vi "NavX_MAIN_2.vi"() -> ()   [LabVIEW 2018]
uses:
  Underlying VI's/NavX VI/navX type def.ctl
  <vilib>/Studica/Studica Toolkit/NavX/TypeDefs/Flags/Z900_navX_Flags_OpStatusTypeDef.ctl
  <vilib>/Studica/Studica Toolkit/NavX/TypeDefs/Flags/Z900_navX_Flags_CalibrationStatusTypeDef.ctl
  <vilib>/Studica/Studica Toolkit/Background/I2C Channel.ctl
  <vilib>/Studica/Studica Toolkit/NavX/NavX.lvlib
panel:
  out "Error Out":errorcluster
  out "Status":T3 {"OP Status" items=["INITIALIZING", "SELFTEST_IN_PROGRESS", "ERROR", "IMU_AUTOCAL_IN_PROGRESS", "NORMAL"]; "Calibration Status" items=["IMU_CAL_STATE_MASK"=3, "IMU_CAL_STATE_INPROGRESS"=0, "IMU_CAL_STATE_ACCUMULATE"=1, "IMU_CAL_STATE_COMPLETE"=2]}
  out "NavX Readings":T4
  in  "Mode":T5=enum."Read Values"
  in  "stop":bool
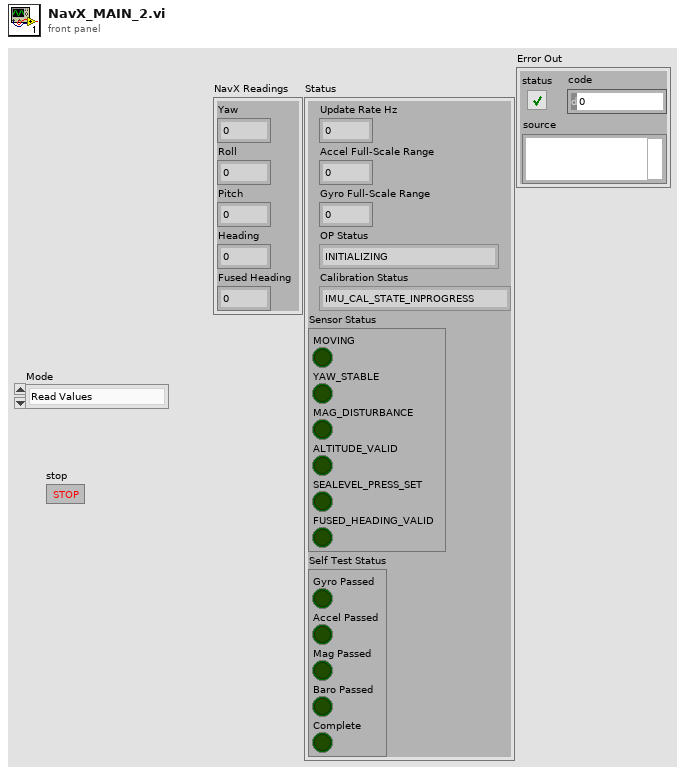
[diagram p1: front panel]
types:
  T1 = typedef "NavX.lvlib/Z900_navX_Flags_OpStatusTypeDef.ctl" = u8
  T2 = typedef "NavX.lvlib/Z900_navX_Flags_CalibrationStatusTypeDef.ctl" = u8
  T3 = cluster{"Update Rate Hz":u8, "Accel Full-Scale Range":u8, "Gyro Full-Scale Range":u16, "OP Status":T1, "Calibration Status":T2, "Sensor Status":cluster{"MOVING":bool, "YAW_STABLE":bool, "MAG_DISTURBANCE":bool, "ALTITUDE_VALID":bool, "SEALEVEL_PRESS_SET":bool, "FUSED_HEADING_VALID":bool}, "Self Test Status":cluster{"Gyro Passed":bool, "Accel Passed":bool, "Mag Passed":bool, "Baro Passed":bool, "Complete":bool}}
  T4 = cluster{"Yaw":dbl, "Roll":dbl, "Pitch":dbl, "Heading":dbl, "Fused Heading":dbl}
  T5 = typedef "navX type def.ctl" = enum16{"Get i2C reference", "Read Values", "Zero Yaw"}
  T6 = typedef "I2C Channel.ctl" = enum16{"Not Connected", "A", "B"}
  T7 = cluster{"I2C Ref Out":cluster{"I2C Channel":T6, "FPGA VI Reference Out":refnum<k20>}, "Connected":bool, "Slave Address (7-bit)":u8, "Registry":u8[]}
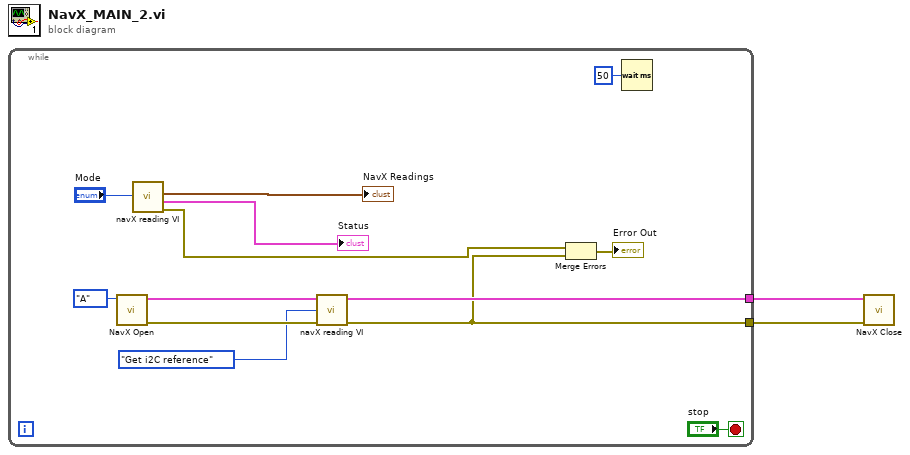
[diagram p0: block diagram]
diagram:
  n1 = while {
    tunnel: [w12] -> w2
    tunnel: [w4] -> w1
    stop <- "stop" stop-if-true
    n2 = call <vilib>:"NavX Open.vi"("I2C Channel"=I2C_Channel."A") -> ("error out"=w13:errorcluster, "NavX Info"=w14:T7)  [unwired: 9 in]
    n3 = call "navX reading VI.vi"("Mode"="Mode") -> ("NavX Readings"=→"NavX Readings":T4, "Status"=→"Status":T3, "Error Out"=w3:errorcluster)  [unwired: 2 in, 1 out]
    n4 = call "navX reading VI.vi"("NavX Info In"=w14, "Mode"=navX_type_def."Get i2C reference", "error in (no error)"=w13) -> ("NavX Info Out"=w12:T7, "Error Out"=w4:errorcluster)  [unwired: 2 out]
    n5 = Merge Errors(w3, w4) -> (→"Error Out":errorcluster)
    n6 = Wait (ms)(milliseconds to wait=u32 50) -> ()  [unwired: 1 out]
  }
  n7 = call <vilib>:"NavX Close.vi"("error in (no error)"=w1, "NavX Info In"=w2) -> ()  [unwired: 9 in, 1 out]
